vi "swapbyte.vi"(4 "SGL 1D":sgl[](array[numeric])=[1.0, 2.0, 3.0, 4.0, 5.0, 6.0, 7.0, 8.0, 9.0, 10.0] format="%.2f", 5 "I32":i32, 6 "I32 1D":i32[](array[numeric])=[1, 2, 3, 4, 5, 6, 7, 8, 9, 10], 7 "SGL":sgl format="%.2f") -> (0 "swapped SGL 1D":sgl[](array[numeric]) format="%.2f", 1 "swapped I32":i32, 2 "swapped I32 1D":i32[](array[numeric]), 3 "swapped SGL":sgl format="%.2f")   [LabVIEW 2013]
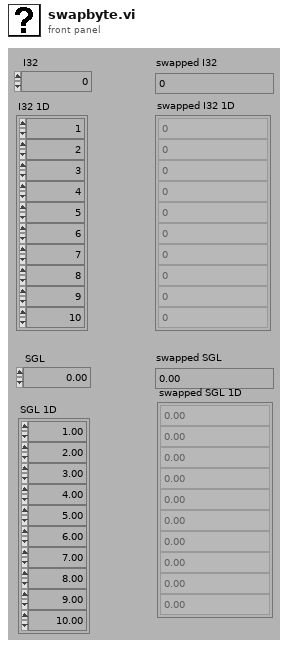
[diagram p1: front panel]
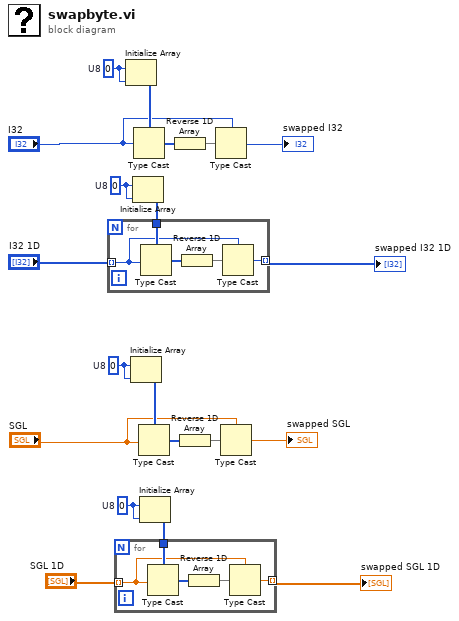
[diagram p0: block diagram]
diagram:
  w4 = u8 0  # U8
  w7 = u8 0  # U8
  w14 = u8 0  # U8
  w20 = u8 0  # U8
  n1 = Initialize Array(w20, w20) -> (w19:u8[])
  n2 = Initialize Array(w14, w14) -> (w13:u8[])
  n3 = Initialize Array(w4, w4) -> (w3:u8[])
  n4 = for {
    tunnel: w3 -> [w24]
    tunnel: [w22] -> w1 mode=indexing
    tunnel: "I32 1D" -> [w21] mode=indexing
    n5 = Type Cast(type=w24, x=w21) -> (*(type *) &x=w25:u8[])
    n6 = Reverse 1D Array(array=w25) -> (reversed array=w23:u8[])
    n7 = Type Cast(type=w21, x=w23) -> (*(type *) &x=w22:i32)
  }
  "swapped I32 1D" <- w1
  n8 = Type Cast(type=w19, x="I32") -> (*(type *) &x=w18:u8[])
  n9 = Type Cast(type=w13, x="SGL") -> (*(type *) &x=w12:u8[])
  n10 = Initialize Array(w7, w7) -> (w6:u8[])
  n11 = for {
    tunnel: w6 -> [w29]
    tunnel: [w27] -> w5 mode=indexing
    tunnel: "SGL 1D" -> [w26] mode=indexing
    n12 = Type Cast(type=w29, x=w26) -> (*(type *) &x=w30:u8[])
    n13 = Reverse 1D Array(array=w30) -> (reversed array=w28:u8[])
    n14 = Type Cast(type=w26, x=w28) -> (*(type *) &x=w27:sgl)
  }
  "swapped SGL 1D" <- w5
  n15 = Reverse 1D Array(array=w18) -> (reversed array=w17:u8[])
  n16 = Reverse 1D Array(array=w12) -> (reversed array=w11:u8[])
  n17 = Type Cast(type="I32", x=w17) -> (*(type *) &x=→"swapped I32":i32)
  n18 = Type Cast(type="SGL", x=w11) -> (*(type *) &x=→"swapped SGL":sgl)
